vi "Mesaje_Oled.vi"() -> ()   [LabVIEW 2023]
uses:
  <vilib>/Instr/_visa.llb/VISA Configure Serial Port (Instr).vi
panel:
  in  "OK Button":bool
  out "String 2":string
  in  "String":string
  in  "stop":bool
  in  "VISA resource name":refnum<visa-resource-name>
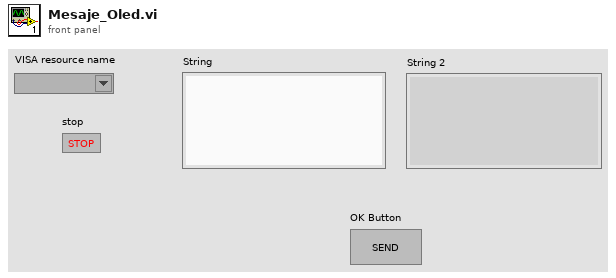
[diagram p1: front panel]
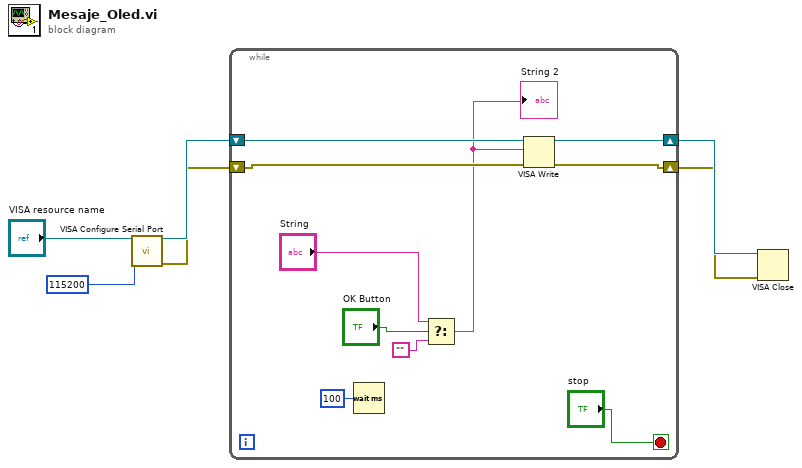
[diagram p0: block diagram]
diagram:
  n1 = call-poly "VISA Configure Serial Port"("VISA resource name"="VISA resource name", "baud rate (9600)"=u32 115200) -> ("VISA resource name out"=w4:refnum<visa-resource-name>, "error out"=w3:errorcluster)  [unwired: 12 in]
  n2 = while {
    shift-right: [w13] -> w2
    shift-left: w4 -> [w15]
    shift-right: [w12] -> w1
    shift-left: w3 -> [w14]
    stop <- "stop" stop-if-true
    n3 = Wait (ms)(milliseconds to wait=u32 100) -> ()  [unwired: 1 out]
    n4 = Select(t="String", s="OK Button", f="") -> (s? t:f=w8:string)
    "String 2" <- w8
    n5 = VISA Write(VISA resource name=w15, write buffer=w8, error in (no error)=w14) -> (VISA resource name out=w13:refnum<visa-resource-name>, error out=w12:errorcluster)  [unwired: 1 out]
  }
  n6 = VISA Close(VISA resource name=w2, error in (no error)=w1) -> ()  [unwired: 1 out]
